vi "Mono10 to U16.vi"(1 "Mono 10 Data":u8[](array[numeric]) format="%08b") -> (0 "U16 Pixels":u16[](array[numeric]) format="%.0b")   [LabVIEW 2020, in "Buffer.lvclass"]
uses:
  Buffer.lvclass
  Buffer.lvclass/Buffer.ctl
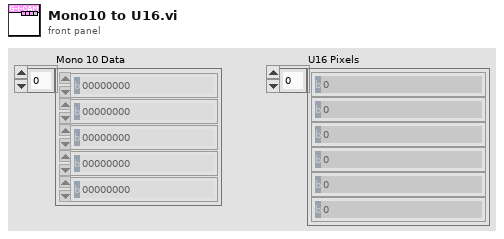
[diagram p1: front panel]
types:
  T1 = enum16{"big-endian, network order", "native, host order", "little-endian"}
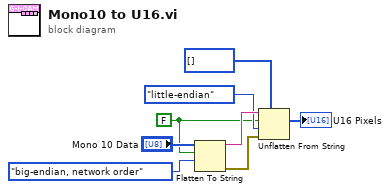
[diagram p0: block diagram]
diagram:
  w2 = FALSE ("prepend array or string size? (T)")
  n1 = Flatten To String(anything="Mono 10 Data", prepend array or string size? (T)=w2, byte order (0:big-endian, network order)=T1."big-endian, network order") -> (data string=w6:string, error out=w1:errorcluster)  [unwired: 1 in, 1 out]
  n2 = Unflatten From String(type=u16[] [] ("unsigned 16bit integer"), binary string=w6, data includes array or string size? (T)=w2, byte order (0:big-endian, network order)=T1."little-endian", error in (no error)=w1) -> (value=→"U16 Pixels":u16[])  [unwired: 2 out]
